vi "testSendEvtFromClient.vi"(8 "error in (no error)":errorcluster) -> (0 "error out":errorcluster)   [LabVIEW 2018]
doc: "This VI sends events from TCP client to TCP server."
uses:
  <vilib>/addons/_JKI Toolkits/Caraya/classes/Assert/Assert Equal Value_Variant.vi
  src/TcpServer/TcpServer.lvclass
  <vilib>/addons/_JKI Toolkits/Caraya/classes/Test/Test.lvclass
  <vilib>/addons/_JKI Toolkits/Caraya/classes/Assert/Assert.lvclass
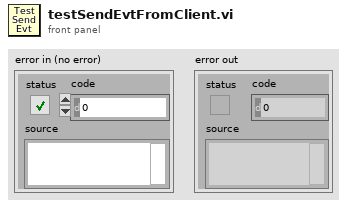
[diagram p1: front panel]
types:
  T1 = cluster{"CmdRead":refnum<user-event>, "EvtRead":refnum<user-event>, "GenRead":refnum<user-event>}
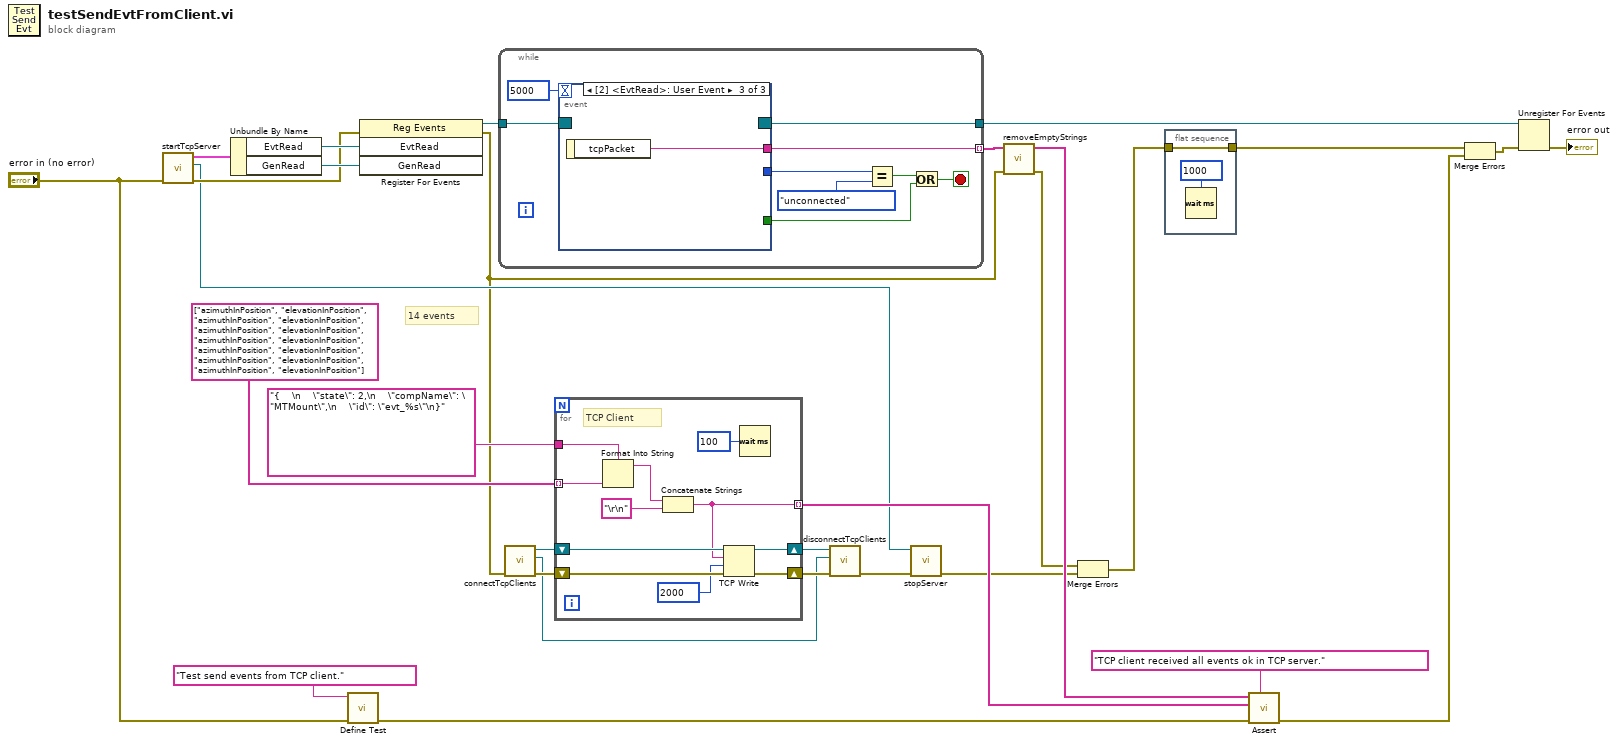
[diagram p0: block diagram]
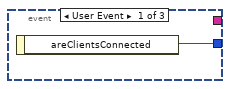
[diagram p2: hidden frame]
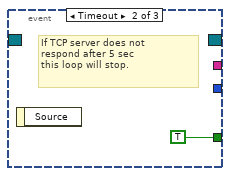
[diagram p3: hidden frame]
diagram:
  # "14 events"
  n1 = call "startTcpServer.vi"("error in (no error)"="error in (no error)") -> ("error out"=w20:errorcluster, "TcpServer out"=w7:refnum<class "TcpServer.lvclass">, "UserEvents"=w24:T1)  [unwired: 8 in]
  n2 = Unbundle By Name(w24) -> ("EvtRead"=w23:refnum<user-event>, "GenRead"=w22:refnum<user-event>)
  n3 = call <vilib>:"Define Test.vi"("error in (no error)"="error in (no error)", "Label (VI Title)"="Test send events from TCP client.") -> ("error out"=w13:errorcluster)  [unwired: 9 in]
  n4 = register-events(error in=w20, w23, w22) -> (reference out=w30:refnum<event-registration>, error out=w4:errorcluster)  [unwired: 1 in]
  n5 = while {
    tunnel: w30 -> [w39]
    tunnel: [w38] -> w29
    tunnel: [w32] -> w6 mode=indexing
    stop <- w33 stop-if-true
    n6 = event shown="[2] <EvtRead>: User Event" {
      selector: w39 -> [_ _ _]
      dyn-events: [_ _ _] -> w38
      timeout: 5000 -> [_ _ _]
      tunnel: [w40 _ _] -> w37
      tunnel: [_ TRUE _] -> w34
      tunnel: [_ _ w42] -> w32
      event User Event {
        n7 = event-data() -> ("areClientsConnected"=w40:enum16{"unchanged", "connected", "unconnected"})  [unwired: 1 in]
      }
      event Timeout {
        # "If TCP server does not\nrespond after 5 sec\nthis loop will stop."
        n8 = event-data() -> ()  [unwired: 1 in, 1 out]
      }
      event User Event {
        n9 = event-data() -> ("tcpPacket"=w42:string)  [unwired: 1 in]
      }
    }
    n10 = Equal?(x=w37, y=enum16{"unchanged", "connected", "unconnected"}."unconnected" ("areClientsConnected")) -> (x = y?=w35:bool)
    n11 = Or(x=w35, y=w34) -> (x .or. y?=w33:bool)
  }
  n12 = call "connectTcpClients.vi"("error in (no error)"=w4) -> ("error out"=w21:errorcluster, "tel connection ID out"=w16:refnum<k5>, "cmd connection ID out"=w27:refnum<k5>)  [unwired: 8 in]
  n13 = for {
    shift-right: [w51] -> w17
    shift-left: w27 -> [w53]
    shift-right: [w50] -> w18
    shift-left: w21 -> [w52]
    tunnel: "{    \n    \"state\": 2,\n    \"compName\": \"MTMount\",\n    \"id\": \"evt_%s\"\n}" ("Display") -> [w49]
    tunnel: string[] ["azimuthInPosition", "elevationInPosition", "azimuthInPosition", "elevationInPosition", "azimuthInPosition", "elevationInPosition", "azimuthInPosition", "elevationInPosition", "azimuthInPosition", "elevationInPosition", "azimuthInPosition", "elevationInPosition", "azimuthInPosition", "elevationInPosition"] -> [w48] mode=indexing
    tunnel: [w43] -> w12 mode=indexing
    # "TCP Client"
    n14 = Format Into String(format string=w49, w48) -> (resulting string=w47:string)  [unwired: 2 in, 1 out]
    n15 = Concatenate Strings(w47, "\r\n" ("string")) -> (w43:string)
    n16 = TCP Write(connection ID=w53, data in=w43, error in (no error)=w52, 9:2000 ("timeout ms (25000)")) -> (connection ID out=w51:refnum<k5>, error out=w50:errorcluster)  [unwired: 1 out]
    n17 = Wait (ms)(milliseconds to wait=u32 100) -> ()  [unwired: 1 out]
  }
  n18 = call "disconnectTcpClients.vi"("error in (no error)"=w18, "tel connection ID in"=w16, "cmd connection ID in"=w17) -> ("error out"=w15:errorcluster)  [unwired: 8 in]
  n19 = call "stopServer.vi"("error in (no error)"=w15, "tcpServer in"=w7) -> ("error out"=w2:errorcluster)  [unwired: 8 in, 1 out]
  n20 = call "removeEmptyStrings.vi"("error in (no error)"=w4, "stringArray in"=w6) -> ("error out"=w3:errorcluster, "stringArray out"=w5:string[])  [unwired: 8 in]
  n21 = Merge Errors(w3, w2) -> (w1:errorcluster)
  n22 = flat-sequence {
    tunnel: w1 -> [w54]
    tunnel: [w54] -> w11
    frame #0 {
      n23 = Wait (ms)(milliseconds to wait=u32 1000) -> ()  [unwired: 1 out]
    }
  }
  n24 = call-poly <vilib>:"Assert.vi"("Label"="TCP client received all events ok in TCP server.", "error in (no error)"=w13, "Y"=w12, "X"=w5) -> ("error out"=w10:errorcluster)  [unwired: 7 in]
  n25 = Merge Errors(w11, w10) -> (w8:errorcluster)
  n26 = Unregister For Events(event registration refnum=w29, error in=w8) -> (error out=→"error out":errorcluster)
